vi "To String.vi"(8 "error in (no error)":errorcluster, 11 "Anytime D* in":refnum<class "NI_Robotics_AnytimeDStar.lvclass">) -> (0 "error out":errorcluster, 2 "output":T1, 3 "Anytime D* out":refnum<class "NI_Robotics_AnytimeDStar.lvclass">)   [LabVIEW 2017, in "NI_Robotics_AnytimeDStar.lvclass"]
uses:
  <vilib>/robotics/Navigation/Anytime D Star/NI_Robotics_AnytimeDStar.lvclass
  <vilib>/robotics/Navigation/Anytime D Star/NI_Robotics_AnytimeDStar.lvclass/NI_Robotics_AnytimeDStar.ctl
  <vilib>/robotics/Navigation/shared/Priority Queue/NI_Robotics_Priority Queue.lvclass
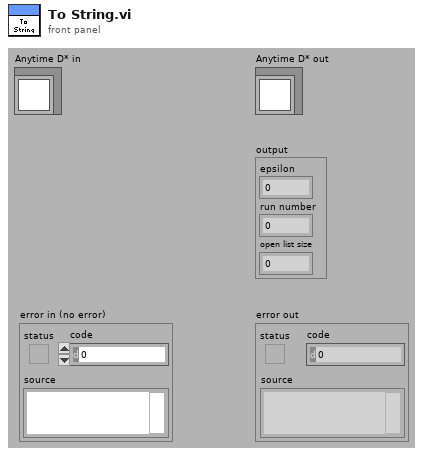
[diagram p1: front panel]
types:
  T1 = cluster{"epsilon":dbl, "run number":i32, "open list size":i32}
  T2 = cluster{"epsilon":dbl, "run number":i32, "num nodes in OPEN":i32}
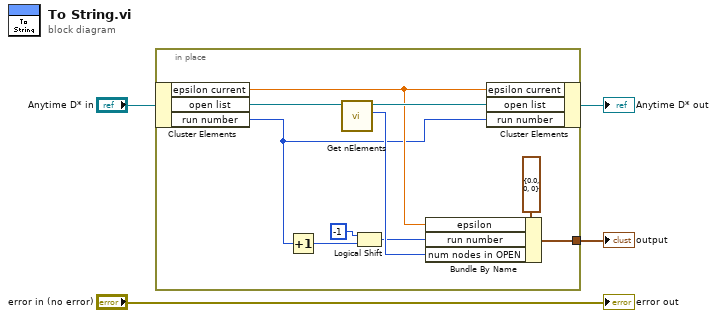
[diagram p0: block diagram]
diagram:
  n1 = in-place {
    in-place-border: [w5] -> w1
    n2 = in-place-cluster #1("Anytime D* in") -> ("epsilon current"=w12:dbl, "open list"=w14:refnum<class "NI_Robotics_Priority Queue.lvclass">, "run number"=w6:i32)
    n3 = Increment(x=w6) -> (x+1=w7:i32)
    n4 = call <vilib>:"Get nElements.vi"("Priority Queue in"=w14) -> ("nElements"=w11:i32, "Priority Queue out"=w13:refnum<class "NI_Robotics_Priority Queue.lvclass">)  [unwired: 9 in]
    n5 = Logical Shift(y=-1 ("x"), x=w7) -> (x << y=w9:i32)
    n6 = Bundle By Name(cluster=T2 {"epsilon"=0.0, "run number"=0, "num nodes in OPEN"=0} ("output 2"), "epsilon"=w12, "run number"=w9, "num nodes in OPEN"=w11) -> (w5:T2)
    n7 = in-place-cluster #1("epsilon current"=w12, "open list"=w13, "run number"=w6) -> (→"Anytime D* out":refnum<class "NI_Robotics_AnytimeDStar.lvclass">)
  }
  "output" <- w1
  "error out" <- "error in (no error)"
